vi "labview_python_send_serial.vi"() -> ()   [LabVIEW 2025]
panel:
  out "Debug":string
  in  "String":string
  in  "baud rate":T1(ring)
  in  "COM port":T2(ring)
  in  "python version":enum16{"3.6", "3.7", "3.8", "3.9", "3.10"}(ring)
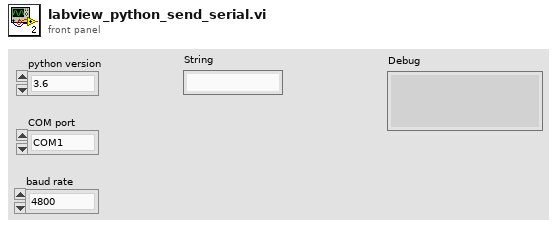
[diagram p1: front panel]
types:
  T1 = enum16{"4800", "9600", "19200", "38400", "57600", "115200"}
  T2 = enum16{"COM1", "COM2", "COM3", "COM4", "COM5", "COM6", "COM7", "COM8", "COM9", "COM10", "COM11", "COM12", "COM13"}
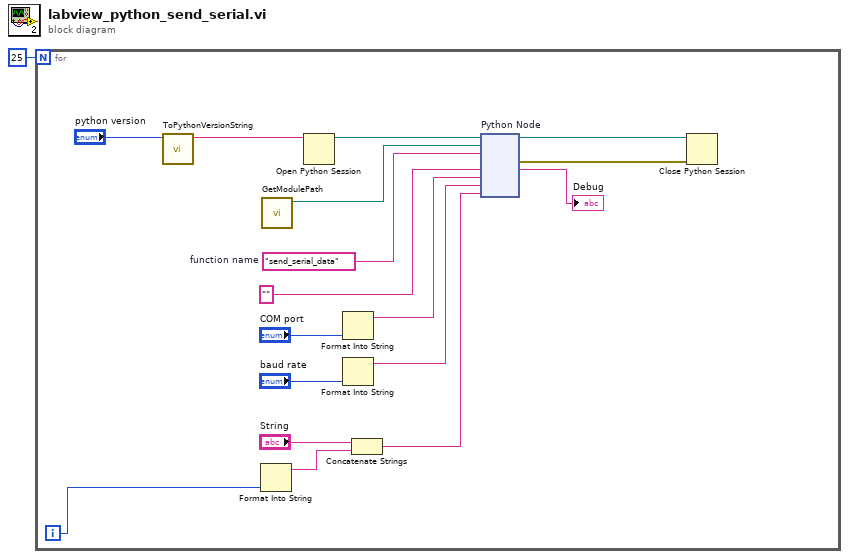
[diagram p0: block diagram]
diagram:
  n1 = for {
    N: 25 -> [_]
    i -> [w7]
    w11 = "send_serial_data"  # function name
    n2 = call "ToPythonVersionString.vi"("python version"="python version") -> ("python version string"=w17:string)  [unwired: 10 in]
    n3 = Format Into String(w7) -> (resulting string=w6:string)  [unwired: 3 in, 1 out]
    n4 = call "GetModulePath.vi"() -> ("module path"=w15:path)  [unwired: 11 in]
    n5 = Open Python Session(python version=w17) -> (session out=w12:refnum<k35>)  [unwired: 2 in, 1 out]
    n6 = Format Into String("COM port") -> (resulting string=w10:string)  [unwired: 3 in, 1 out]
    n7 = Format Into String("baud rate") -> (resulting string=w8:string)  [unwired: 3 in, 1 out]
    n8 = Concatenate Strings("String", w6) -> (w4:string)
    n9 = node "Python Node"(w12, w15, w11, "", w10, w8, w4) -> (w13:refnum<k35>, w14:errorcluster, →"Debug":string)  [unwired: 4 in, 2 out]
    n10 = Close Python Session(session in=w13, error in=w14) -> ()  [unwired: 1 out]
  }
